vi "counterTool_pend.vi"(0 "Counts":dbl, 1 "Pendulum Scale":dbl=1079.0, 2 "Zero":bool, 4 "Output Units":enum16{"Degrees", "Radians"}(ring)) -> (6 "Total Angle":dbl=72.0, 7 "Wrap Angle":dbl)   [LabVIEW 2025]
doc: "Voltage - Input voltage value\nDeg/Volt - Constant multiplier to convert input voltage to angular value\n\nTotal Angle - Current accumulated angle -Inf to Inf degrees\nWrap Angle - Current angle 0 to 360 degrees"
panel:
  out "Cycles":dbl
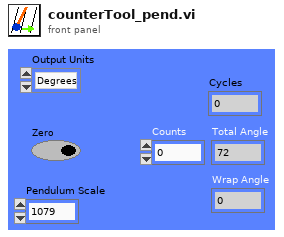
[diagram p1: front panel]
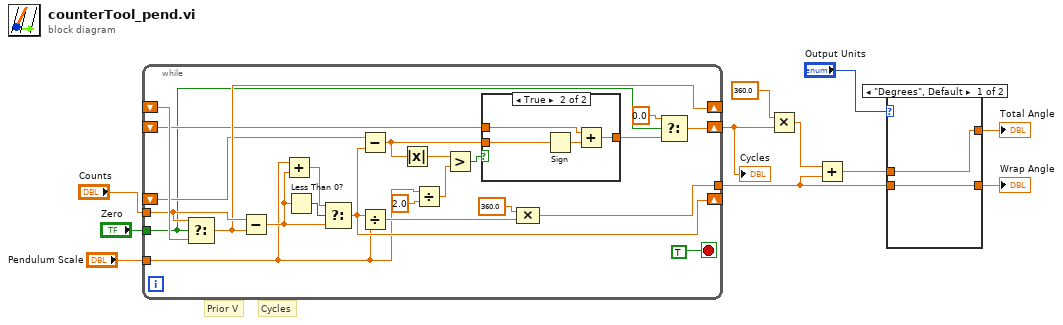
[diagram p0: block diagram]
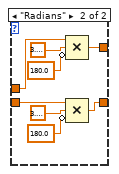
[diagram p2: hidden frame]
diagram:
  # "Prior V"
  # "Cycles"
  n1 = while {
    tunnel: [w24] -> w3
    shift-right: [w27] -> w10
    shift-left: _ -> [w16]
    tunnel: "Counts" -> [w22]
    shift-right: [w17] -> _
    shift-left: _ -> [w15]
    tunnel: "Zero" -> [w14]
    shift-right: [w21] -> _
    shift-left: _ -> [w23]
    tunnel: "Pendulum Scale" -> [w12]
    stop <- TRUE stop-if-true
    n2 = Select(t=w22, s=w14, f=w23) -> (s? t:f=w21:dbl)
    n3 = Subtract(x=w22, y=w21) -> (x-y=w18:dbl)
    n4 = Add(x=w12, y=w18) -> (x+y=w19:dbl)
    n5 = Less Than 0?(x=w18) -> (x < 0?=w20:bool)
    n6 = Select(t=w19, s=w20, f=w18) -> (s? t:f=w17:dbl)
    n7 = Subtract(x=w15, y=w17) -> (x-y=w31:dbl)
    n8 = Divide(x=w17, y=w12) -> (x/y=w28:dbl)
    n9 = Absolute Value(x=w31) -> (abs(x)=w33:dbl)
    n10 = Divide(x=w12, y=2.0) -> (x/y=w29:dbl)
    n11 = Greater?(x=w33, y=w29) -> (0:w32:bool)
    n12 = case shown="True" w32 {
      tunnel: [w35 w39] -> w26
      tunnel: w16 -> [w35 w38]
      tunnel: w31 -> [_ w37]
      frame False {
      }
      frame True {
        n13 = Sign(1:w37) -> (0:w36:dbl)
        n14 = Add(x=w38, y=w36) -> (x+y=w39:dbl)
      }
    }
    n15 = Compound Arithmetic op=MULTIPLY(360.0 ("y"), w28) -> (w24:dbl)
    n16 = Select(t=0.0, s=w14, f=w26) -> (s? t:f=w27:dbl)
  }
  "Cycles" <- w10
  n17 = Multiply(x=360.0 ("y"), y=w10) -> (x*y=w11:dbl)
  n18 = Add(x=w11, y=w3) -> (x+y=w5:dbl)
  n19 = case shown="\"Degrees\", Default" "Output Units" {
    tunnel: [w41 w47] -> w4
    tunnel: w5 -> [w41 w46]
    tunnel: w3 -> [w40 w43]
    tunnel: [w40 w42] -> w2
    frame "Degrees", Default {
    }
    frame "Radians" {
      n20 = Compound Arithmetic op=MULTIPLY(w46, 3.141592653589793, invert 180.0 ("value")) -> (w47:dbl)
      n21 = Compound Arithmetic op=MULTIPLY(w43, 3.141592653589793, invert 180.0 ("value")) -> (w42:dbl)
    }
  }
  "Wrap Angle" <- w2
  "Total Angle" <- w4
